vi "retrieve_trace_example.vi"() -> ()   [LabVIEW 2020, in "Data.PG.lvclass"]
uses:
  Data.PG.lvclass
panel:
  in  "max points":i32
  out "XY Graph":cluster{timestamp[], dbl[]}(graph)
  in  "path table:column":string
  in  "End":timestamp
  in  "Start":timestamp
  out "Data.PG out":refnum<class "Data.PG.lvclass">
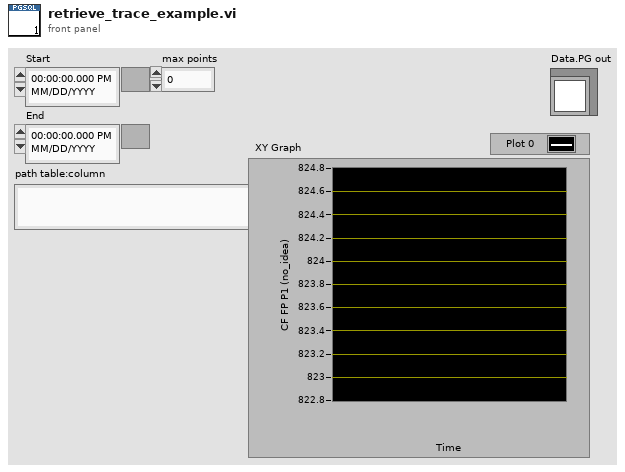
[diagram p1: front panel]
types:
  T1 = cluster{"host":string, "port":string, "dbname":string, "user":string, "password":string}
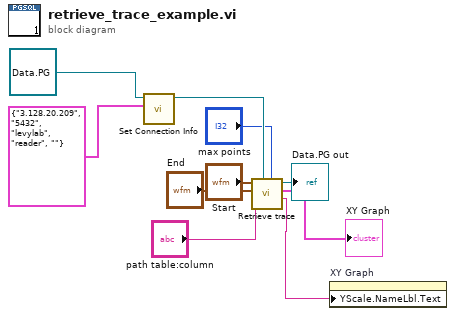
[diagram p0: block diagram]
diagram:
  n1 = call "Set Connection Info.vi"("connection info"=T1 {"host"="3.128.20.209", "port"="5432", "dbname"="levylab", "user"="reader", "password"=""}, "Data.PG in"=refnum<class "Data.PG.lvclass"> refnum) -> ("Data.PG out"=w8:refnum<class "Data.PG.lvclass">)  [unwired: 8 in, 1 out]
  n2 = call "Retrieve trace.vi"("max points"="max points", "Data.PG in"=w8, "path table:column"="path table:column", "End"="End", "Start"="Start") -> ("Column (units)"=w1:string, "Trace"=→"XY Graph":cluster{timestamp[], dbl[]}, "Data.PG out"=→"Data.PG out":refnum<class "Data.PG.lvclass">)  [unwired: 3 in, 1 out]
  n3 = property on="XY Graph" class="XYGraph (strict)"("YScale.NameLbl.Text"=w1) -> ()  [unwired: 2 in, 2 out]
